vi "Shooter Tele-Op.vi"(8 "POVs":i16[](array[numeric]), 9 "Buttons":bool[](array[boolean]), 10 "Axes":dbl[](array[numeric])) -> ()   [LabVIEW 2019]
uses:
  Implementation/Shooter Operations.ctl
  fabf2f16-a199-41ce-a1f9-928ef0d5b822.vi
  f3a45681-08c3-4dc6-9d07-57e32a89152a.vi
  61e2efad-2388-46bd-aca9-edd97e37118f.vi
  eb2ad1ab-fb17-4d60-b788-7adaa2e38171.vi
panel:
  in  "Down?":bool
  in  "Zone 1":cluster{dbl, dbl}={4500.0, 14.5}
  in  "Zone 2":cluster{dbl, dbl}={3850.0, 10.5}
  in  "Zone 4":cluster{dbl, dbl}={5350.0, 18.4}
  in  "Zone 3":cluster{dbl, dbl}={4500.0, 14.0}
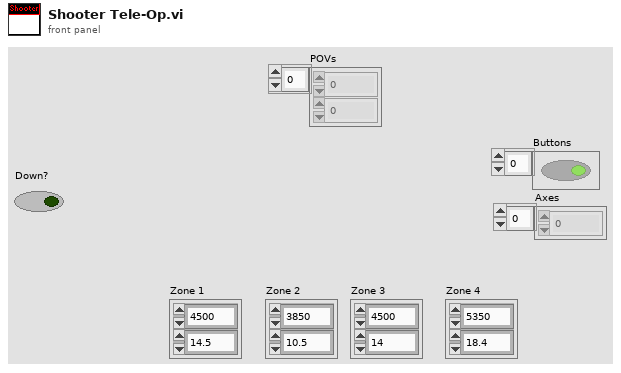
[diagram p1: front panel]
types:
  T1 = typedef "Shooter Operations.ctl" = enum16{"Reserve", "Read Current", "Immediate", "Shoot"}
  T2 = cluster{"f":dbl, "upper limit":dbl, bool, "upper limit":dbl}
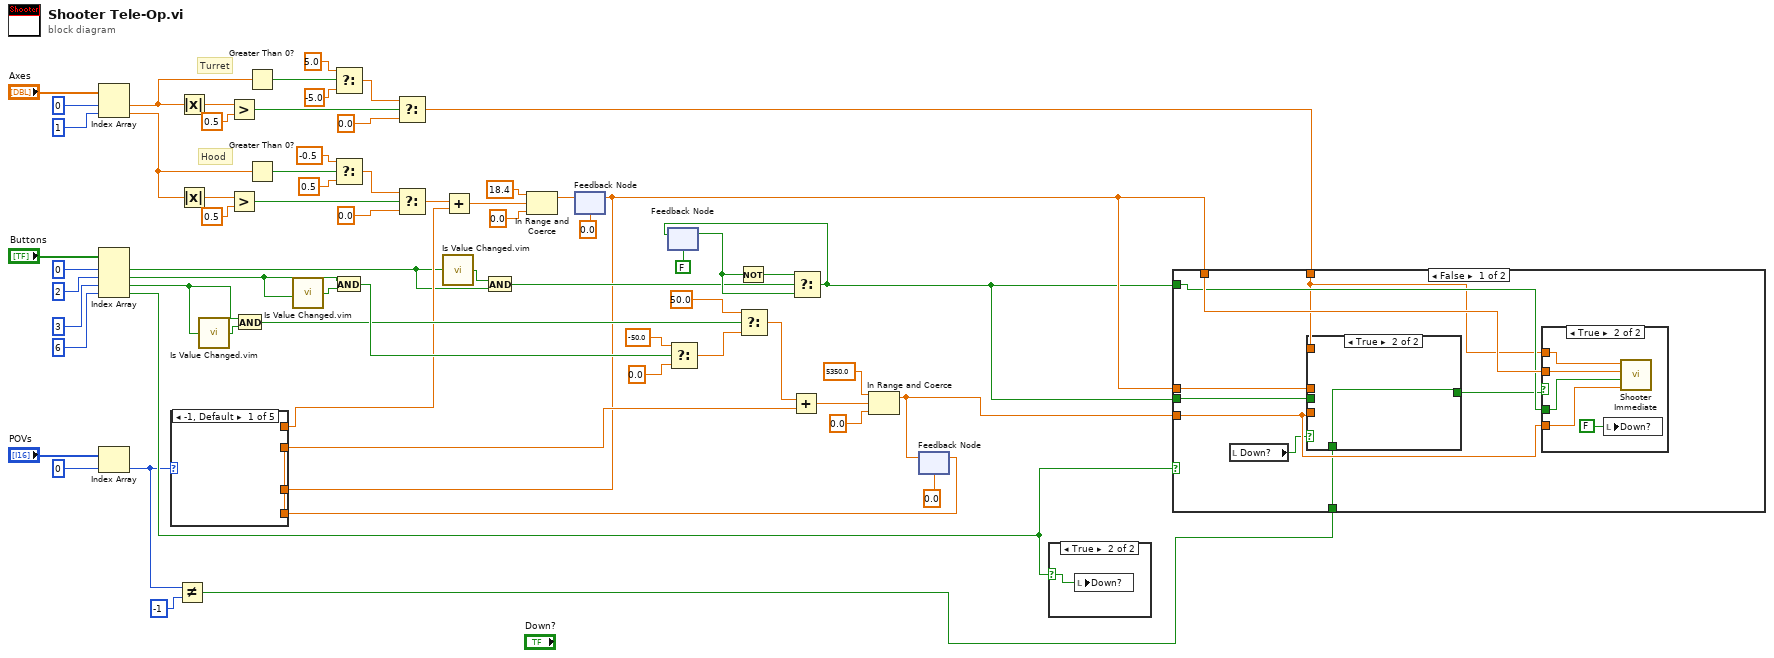
[diagram p0: block diagram]
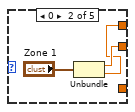
[diagram p3: hidden frame]
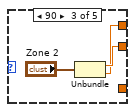
[diagram p4: hidden frame]
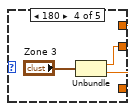
[diagram p5: hidden frame]
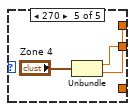
[diagram p6: hidden frame]
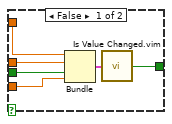
[diagram p7: hidden frame]
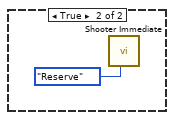
[diagram p9: hidden frame]
diagram:
  # "Turret"
  # "Hood"
  n1 = Index Array(array="Axes", index #1=0 ("index"), index #2=1 ("index")) -> (element #1=w50:dbl, element #2=w54:dbl)
  n2 = Index Array(array="Buttons", index #1=0 ("index"), index #2=2 ("X"), index #3=3 ("Y"), index #4=6 ("Menu")) -> (element #1=w10:bool, element #2=w23:bool, element #3=w11:bool, element #4=w4:bool)
  n3 = Index Array(array="POVs", index=0) -> (element=w3:i16)
  n4 = Not Equal?(x=w3, y=i16 -1) -> (x != y?=w1:bool)
  n5 = Absolute Value(x=w50) -> (abs(x)=w33:dbl)
  n6 = Absolute Value(x=w54) -> (abs(x)=w57:dbl)
  n7 = call "Is Value Changed.vim"("value"=w11) -> ("changed or first call?"=w25:bool)
  n8 = Greater?(x=w33, y=0.5) -> (0:w31:bool)
  n9 = Greater?(x=w57, y=0.5) -> (0:w55:bool)
  n10 = And(x=w11, y=w25) -> (x .and. y?=w21:bool)
  n11 = Greater Than 0?(x=w50) -> (x > 0?=w29:bool)
  n12 = Greater Than 0?(x=w54) -> (x > 0?=w53:bool)
  n13 = call "Is Value Changed.vim"("value"=w23) -> ("changed or first call?"=w24:bool)
  n14 = Select(t=5.0, s=w29, f=-5.0) -> (s? t:f=w26:dbl)
  n15 = Select(t=-0.5, s=w53, f=0.5) -> (s? t:f=w49:dbl)
  n16 = And(x=w23, y=w24) -> (x .and. y?=w22:bool)
  n17 = Select(t=w26, s=w31, f=0.0) -> (s? t:f=w12:dbl)
  n18 = Select(t=w49, s=w55, f=0.0) -> (s? t:f=w48:dbl)
  n19 = call "Is Value Changed.vim"("value"=w10) -> ("changed or first call?"=w15:bool)
  n20 = And(x=w15, y=w10) -> (x .and. y?=w16:bool)
  n21 = feedback #1(0.0 ("upper limit")) -> (w7:dbl)
  n22 = feedback #2(FALSE) -> (w17:bool)
  n23 = Select(t=-50.0 ("t 2"), s=w22, f=0.0) -> (s? t:f=w45:dbl)
  n24 = Not(x=w17) -> (.not. x?=w18:bool)
  n25 = Select(t=50.0, s=w21, f=w45) -> (s? t:f=w41:dbl)
  n26 = Select(t=w18, s=w16, f=w17) -> (s? t:f=w6:bool)
  n27 = feedback-in #2(w6) -> ()
  n28 = feedback #3(0.0 ("upper limit")) -> (w60:dbl)
  n29 = case shown="-1, Default" w3 {
    tunnel: [w67 w70 w73 w76 w79] -> w8
    tunnel: w60 -> [w67 _ _ _ _]
    tunnel: [w68 w69 w72 w75 w78] -> w13
    tunnel: w7 -> [w68 _ _ _ _]
    frame -1, Default {
    }
    frame 0 {
      n30 = Unbundle("Zone 1") -> (w70:dbl, w69:dbl)
    }
    frame 90 {
      n31 = Unbundle("Zone 2") -> (w73:dbl, w72:dbl)
    }
    frame 180 {
      n32 = Unbundle("Zone 3") -> (w76:dbl, w75:dbl)
    }
    frame 270 {
      n33 = Unbundle("Zone 4") -> (w79:dbl, w78:dbl)
    }
  }
  n34 = Add(x=w48, y=w13) -> (x+y=w37:dbl)
  n35 = In Range and Coerce(upper limit=18.4, x=w37, lower limit=0.0) -> (coerced(x)=w14:dbl)  [unwired: 1 out]
  n36 = feedback-in #1(w14) -> ()
  n37 = Add(x=w41, y=w8) -> (x+y=w40:dbl)
  n38 = In Range and Coerce(upper limit=5350.0, x=w40, lower limit=0.0) -> (coerced(x)=w5:dbl)  [unwired: 1 out]
  n39 = feedback-in #3(w5) -> ()
  n40 = case shown="True" w4 {
    selector: w4 -> [_ w81]
    frame False {
    }
    frame True {
      n41 = local write "Down?"(w81) -> ()
    }
  }
  n42 = case shown="False" w4 {
    tunnel: w12 -> [w88 _]
    tunnel: w7 -> [w90 _]
    tunnel: w6 -> [w89 _]
    tunnel: w5 -> [w85 _]
    tunnel: w7 -> [w87 _]
    tunnel: w6 -> [w86 _]
    tunnel: w1 -> [w82 _]
    frame False {
      n43 = local read "Down?"() -> (w84:bool)
      n44 = case shown="True" w84 {
        tunnel: w88 -> [w95 _]
        tunnel: w87 -> [w94 _]
        tunnel: w86 -> [w93 _]
        tunnel: w85 -> [w92 _]
        tunnel: [w91 w97] -> w83
        tunnel: w82 -> [_ w97]
        frame False {
          n45 = Bundle("f"=w95, "upper limit"=w94, w93, "upper limit"=w92) -> (w96:T2)  [unwired: 1 in]
          n46 = call "Is Value Changed.vim"("value"=w96) -> ("changed or first call?"=w91:bool)
        }
        frame True {
        }
      }
      n47 = case shown="True" w83 {
        tunnel: w90 -> [_ w101]
        tunnel: w88 -> [_ w102]
        tunnel: w89 -> [_ w100]
        tunnel: w85 -> [_ w99]
        frame False {
        }
        frame True {
          n48 = local write "Down?"(FALSE ("Down?")) -> ()
          n49 = call "Shooter Immediate.vi"("Flywheel"=w99, "AA?"=w100, "Hood"=w101, "Manual Addition"=w102) -> ()  [unwired: 8 in]
        }
      }
    }
    frame True {
      n50 = call "Shooter Immediate.vi"("Operation"=Shooter_Operations."Reserve") -> ()  [unwired: 11 in]
    }
  }
